vi "angle global.vi"() -> ()   [LabVIEW 2019]
panel:
  in  "angle":dbl
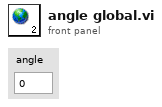
[diagram p1: front panel]
diagram:
